vi "Parse Player Data.vi"(11 "Remaining String in":string) -> (0 "Remaining String out":string, 3 "Player Data":string[](array[string]))   [LabVIEW 2020]
uses:
  <vilib>/regexp/Match Regular Expression.xnode
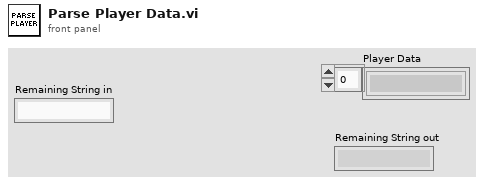
[diagram p1: front panel]
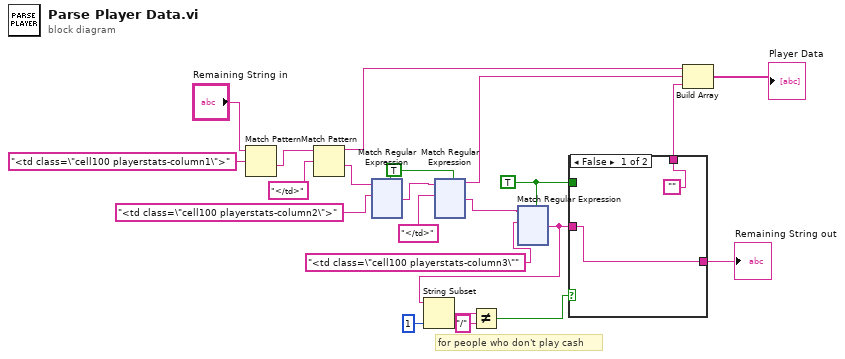
[diagram p0: block diagram]
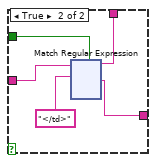
[diagram p2: hidden frame]
diagram:
  w21 = TRUE ("multiline? (F)")
  w19 = TRUE ("multiline? (F)")
  # "for people who don't play cash"
  n1 = Match Pattern(string="Remaining String in", regular expression="<td class=\"cell100 playerstats-column1\">") -> (after substring=w14:string)  [unwired: 1 in, 3 out]
  n2 = Match Pattern(string=w14, regular expression="</td>") -> (before substring=w4:string, after substring=w17:string)  [unwired: 1 in, 2 out]
  n3 = xnode "Match Regular Expression"("input string"=w17, "regular expression"="<td class=\"cell100 playerstats-column2\">", "multiline? (F)"=w19) -> ("after match"=w18:string)  [unwired: 3 in, 4 out]
  n4 = xnode "Match Regular Expression"("input string"=w18, "regular expression"="</td>", "multiline? (F)"=w19) -> ("before match"=w3:string, "after match"=w20:string)  [unwired: 3 in, 3 out]
  n5 = xnode "Match Regular Expression"("input string"=w20, "regular expression"="<td class=\"cell100 playerstats-column3\"", "multiline? (F)"=w21) -> ("after match"=w9:string)  [unwired: 3 in, 4 out]
  n6 = String Subset(string=w9, length (rest)=1 ("length (rest)")) -> (substring=w7:string)  [unwired: 1 in]
  n7 = Not Equal?(x=w7, y="/") -> (x != y?=w5:bool)
  n8 = case shown="False" w5 {
    tunnel: [w23 w29] -> w22
    tunnel: w21 -> [_ w28]
    tunnel: w9 -> [w23 w27]
    tunnel: ["" w26] -> w2
    frame False {
    }
    frame True {
      n9 = xnode "Match Regular Expression"("input string"=w27, "regular expression"="</td>", "multiline? (F)"=w28) -> ("before match"=w26:string, "after match"=w29:string)  [unwired: 3 in, 3 out]
    }
  }
  "Remaining String out" <- w22
  n10 = Build Array(w4, w3, w2) -> (→"Player Data":string[])
